vi "Add Plugin with Children.vi"(7 "Plugin configuration":T1={"name"="", "components"=[], "cycle timing"={"priority"=100, "decimation"=1, "offset"=0}, "threads"=[], "Transfer Groups"=[], "settings"=[]} {"Transfer Groups"."Transfers"."channels"."string offset" format="%d bytes"}, 8 "error in (no error)":errorcluster, 9 "Plugin":refnum<class "Plugin.lvclass">, 10 "parent tag":string, 11 "Application Data In":T12) -> (0 "error out":errorcluster, 2 "average bandwidth":dbl, 3 "Application Data Out":T12)   [LabVIEW 2017, in "DSF Core.lvlib"]
uses:
  DSF Core.lvlib
  Main VI/Application Data.ctl
  LabVIEW-Memory/Source/Classes/Pointer/Pointer.lvclass
  Classes/Framework/Framework.lvclass
  Buffer Reader/Buffer Data.ctl
  Classes/Buffer/Buffer.lvclass
  C:/Git/DSF/LabVIEW-Memory/Source/Classes/Pointer/Pointer.lvclass
  Classes/Transfer Group Status/Status.lvclass
  Typedefs/DSF Data Type.ctl
  Typedefs/DSF Engine Channel Configuration.ctl
  Typedefs/DSF Settings Info.ctl
  Typedefs/DSF Byte Order.ctl
  Typedefs/DSF Engine Framework Configuration.ctl
  Typedefs/DSF Engine Plugin Configuration.ctl
  Typedefs/DSF Timing Info.ctl
  Typedefs/DSF Engine Plugin Thread Configuration.ctl
  Typedefs/DSF Engine Transfer Group Configuration.ctl
  Typedefs/DSF Direction.ctl
  Typedefs/DSF Engine Transfer Configuration.ctl
  Typedefs/DSF Timeout Behavior.ctl
  Classes/Plugin/Plugin.lvclass
  Classes/Plugin/Plugin.lvclass/Plugin.ctl
  Classes/Timing/Timing.lvclass/Timing.ctl
  ID to Tree Items/Tree Item Type.ctl
  Classes/Transfer Group/Transfer Group.lvclass/Transfer Group.ctl
  Classes/Buffers/Buffers.lvclass/Buffers.ctl
  Classes/Transfer/Transfer.lvclass/Transfer.ctl
  Add Transfer with Children.vi
  Classes/Transfer Group/Get Transfers.vi
  Classes/Transfer Group/Get Inline.vi
  Buffer Reader/Average Cycle Bandwidth.vi
  Classes/Transfer Group/Get ID.vi
  Add Buffers with Children.vi
  Classes/Buffer/Get Buffer Size.vi
  Classes/Buffers/Get Inline Buffer.vi
  Classes/Buffers/Get Async Buffer.vi
  Add Buffer Channels.vi
  Sizeof.vi
  LabVIEW-Memory/Source/Classes/Pointer/Get Size.vi
  Classes/Buffer/Subset Buffer.vi
  Classes/Timing/Timing.lvclass
  Classes/Buffers/Buffers.lvclass
  Classes/Transfer Group/Transfer Group.lvclass
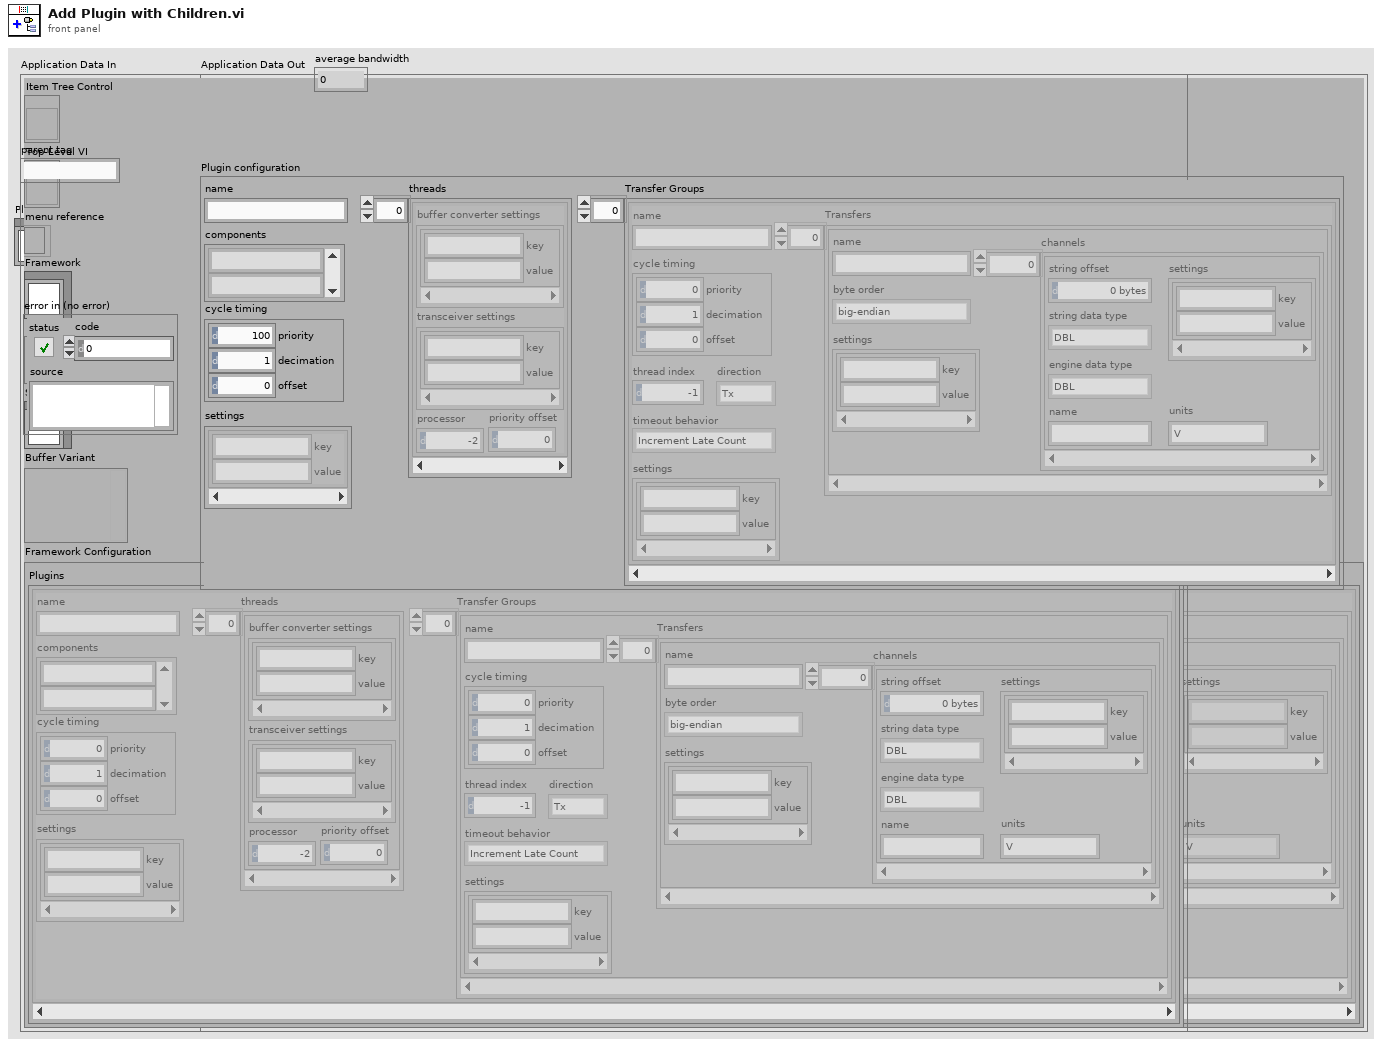
[diagram p1: front panel]
types:
  T1 = typedef "DSF Core.lvlib/DSF Engine Plugin Configuration.ctl" = cluster{"name":string, "components":string[], "cycle timing":T2, "threads":T3[], "Transfer Groups":T5[], "settings":T4}
  T2 = typedef "DSF Core.lvlib/DSF Timing Info.ctl" = cluster{"priority":u64, "decimation":u64, "offset":u64}
  T3 = typedef "DSF Core.lvlib/DSF Engine Plugin Thread Configuration.ctl" = cluster{"buffer converter settings":T4, "transceiver settings":T4, "processor":i32, "priority offset":i16}
  T4 = typedef "DSF Core.lvlib/DSF Settings Info.ctl" = cluster{"key":string, "value":string}[]
  T5 = typedef "DSF Core.lvlib/DSF Engine Transfer Group Configuration.ctl" = cluster{"name":string, "direction":T6, "cycle timing":T2, "thread index":i32, "settings":T4, "Transfers":T7[], "timeout behavior":T11}
  T6 = typedef "DSF Core.lvlib/DSF Direction.ctl" = enum8{"Tx", "Rx"}
  T7 = typedef "DSF Core.lvlib/DSF Engine Transfer Configuration.ctl" = cluster{"name":string, "byte order":T8, "settings":T4, "channels":T9[]}
  T8 = typedef "DSF Core.lvlib/DSF Byte Order.ctl" = enum8{"big-endian", "little-endian"}
  T9 = typedef "DSF Core.lvlib/DSF Engine Channel Configuration.ctl" = cluster{"string offset":u64, "string data type":T10, "engine data type":T10, "name":string, "settings":T4, "units":string}
  T10 = typedef "DSF Core.lvlib/DSF Data Type.ctl" = enum8{"Bool", "SGL", "DBL", "I8", "I16", "I32", "I64", "U8", "U16", "U32", "U64"}
  T11 = typedef "DSF Core.lvlib/DSF Timeout Behavior.ctl" = enum8{"Increment Late Count", "Throw Error"}
  T12 = typedef "DSF Core.lvlib/Application Data.ctl" = cluster{"Item Tree Control":refnum<vi>, "Top-Level VI":refnum<vi>, "menu reference":refnum<k9>, "Framework":refnum<class "Framework.lvclass">, "buffer queue":refnum<queue>, "Stop Pointer":refnum<class "Pointer.lvclass">, "Buffer Variant":variant, "Framework Configuration":T13}
  T13 = typedef "DSF Core.lvlib/DSF Engine Framework Configuration.ctl" = cluster{"Plugins":T1[]}
  T14 = typedef "DSF Core.lvlib/Buffer Data.ctl" = cluster{"Buffer":refnum<class "Buffer.lvclass">, "Status":refnum<class "Status.lvclass">, "decimation":u64, "avg bandwidth":dbl, "data type":T10, "units":string, "channels":T9[], "channel":bool, "engine (T) / string (F)":bool, "byte order":T8}
  T15 = typedef "DSF Core.lvlib/Tree Item Type.ctl" = enum16{"Framework", "Plugin Group", "Plugin", "Group", "Transfer", "Buffer", "Channel"}
  T16 = typedef "DSF Core.lvlib/Tree Item.ctl" = cluster{"Left Cell String":string, "Child Text":string[], "Child Tag":string, "Glyph Index":i32}
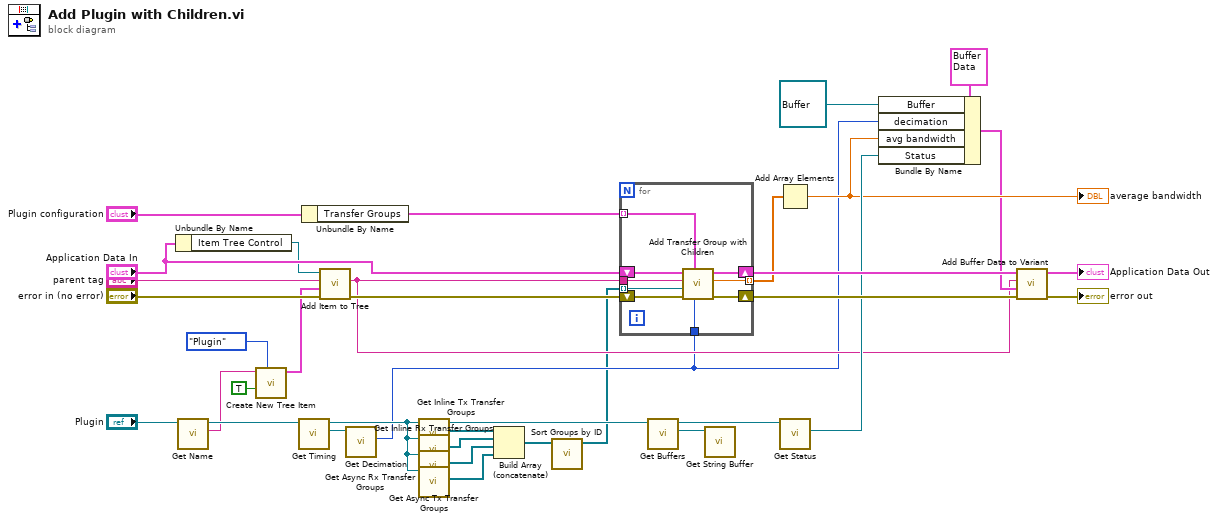
[diagram p0: block diagram]
diagram:
  n1 = Unbundle By Name("Application Data In") -> ("Item Tree Control"=w18:refnum<vi>)
  n2 = call "Get Name.vi"("Plugin in"="Plugin") -> ("name"=w16:string, "Plugin out"=w17:refnum<class "Plugin.lvclass">)  [unwired: 9 in]
  n3 = call "Create New Tree Item.vi"("Item Type"=Tree_Item_Type."Plugin", "found?"=TRUE, "Left Cell String"=w16) -> ("Item"=w31:T16)  [unwired: 7 in, 1 out]
  n4 = call "Get Timing.vi"("Plugin in"=w17) -> ("Timing"=w24:refnum<class "Timing.lvclass">, "Plugin out"=w13:refnum<class "Plugin.lvclass">)  [unwired: 9 in]
  n5 = Unbundle By Name("Plugin configuration") -> ("Transfer Groups"=w8:T5[])
  n6 = call "Add Item to Tree.vi"("error in (no error)"="error in (no error)", "Item"=w31, "parent tag"="parent tag", "TreeControl in"=w18) -> ("error out"=w25:errorcluster, "new item tag"=w3:string)  [unwired: 5 in, 1 out]
  n7 = call "Get Decimation.vi"("Timing in"=w24) -> ("Decimation"=w2:u64)  [unwired: 9 in, 1 out]
  n8 = call "Get Inline Tx Transfer Groups.vi"("Plugin in"=w13) -> ("Inline Tx Transfer Groups"=w14:refnum<class "Transfer Group.lvclass">[], "Plugin out"=w32:refnum<class "Plugin.lvclass">)  [unwired: 9 in]
  n9 = call "Get Inline Rx Transfer Groups.vi"("Plugin in"=w13) -> ("Inline Rx Transfer Groups"=w12:refnum<class "Transfer Group.lvclass">[])  [unwired: 9 in, 1 out]
  n10 = call "Get Async Tx Transfer Groups.vi"("Plugin in"=w13) -> ("Async Tx Transfer Groups"=w11:refnum<class "Transfer Group.lvclass">[])  [unwired: 9 in, 1 out]
  n11 = call "Get Async Rx Transfer Groups.vi"("Plugin in"=w13) -> ("Async Rx Transfer Groups"=w10:refnum<class "Transfer Group.lvclass">[])  [unwired: 9 in, 1 out]
  n12 = Build Array (concatenate)(w14, w12, w11, w10) -> (w9:refnum<class "Transfer Group.lvclass">[])
  n13 = call "Sort Groups by ID.vi"("Transfers Groups in"=w9) -> ("ID-sorted Transfers Groups out"=w1:refnum<class "Transfer Group.lvclass">[])  [unwired: 9 in, 1 out]
  n14 = for {
    tunnel: w3 -> [w40]
    tunnel: w1 -> [w41] mode=indexing
    shift-right: [w42] -> w30
    shift-left: "Application Data In" -> [w45]
    shift-right: [w43] -> w29
    shift-left: w25 -> [w44]
    tunnel: [w38] -> w5 mode=indexing
    tunnel: w8 -> [w37] mode=indexing
    tunnel: w2 -> [w39]
    # "Inline Tx Groups"
    n15 = call "Add Transfer Group with Children.vi"("Plugin Decimation (1)"=w39, "Transfer Group configuration"=w37, "error in (no error)"=w44, "Transfer Group"=w41, "parent tag"=w40, "Application Data In"=w45) -> ("error out"=w43:errorcluster, "average bandwidth"=w38:dbl, "Application Data In"=w42:T12)  [unwired: 3 in]
  }
  n16 = call "Get Buffers.vi"("Plugin in"=w32) -> ("Buffers"=w26:refnum<class "Buffers.lvclass">, "Plugin out"=w21:refnum<class "Plugin.lvclass">)  [unwired: 9 in]
  n17 = call "Get String Buffer.vi"("Buffers in"=w26) -> ()  [unwired: 9 in, 2 out]
  n18 = Add Array Elements(numeric array=w5) -> (sum=w7:dbl)
  "average bandwidth" <- w7
  n19 = call "Get Status.vi"("Plugin in"=w21) -> ("status pointer"=w20:refnum<class "Status.lvclass">)  [unwired: 9 in, 1 out]
  n20 = Bundle By Name(cluster=T14 {"Buffer"=refnum, "Status"=refnum, "decimation"=0, "avg bandwidth"=0.0, "data type"=enum."Bool", "units"="", "channels"=[], "channel"=FALSE, "engine (T) / string (F)"=FALSE, "byte order"=enum."little-endian"} ("Buffer data"), "Buffer"=refnum<class "Buffer.lvclass"> refnum, "decimation"=w2, "avg bandwidth"=w7, "Status"=w20) -> (w4:T14)
  n21 = call "Add Buffer Data to Variant.vi"("error in (no error)"=w29, "Buffer data"=w4, "tag"=w3, "Application Data In in"=w30) -> ("error out"=→"error out":errorcluster, "Application Data In out"=→"Application Data Out":T12)  [unwired: 6 in]
